vi "Close.vi"(8 "error in (no error)":errorcluster, 11 "Diode IV in":refnum<class "Diode IV.lvclass">) -> (0 "error out":errorcluster, 3 "Diode IV out":refnum<class "Diode IV.lvclass">)   [LabVIEW 2015, in "Diode Characterization.lvlib" / "Diode IV.lvclass"]
uses:
  Diode IV.lvclass
  <userlib>/Common Components/Measurement Actor/Measurement.lvclass
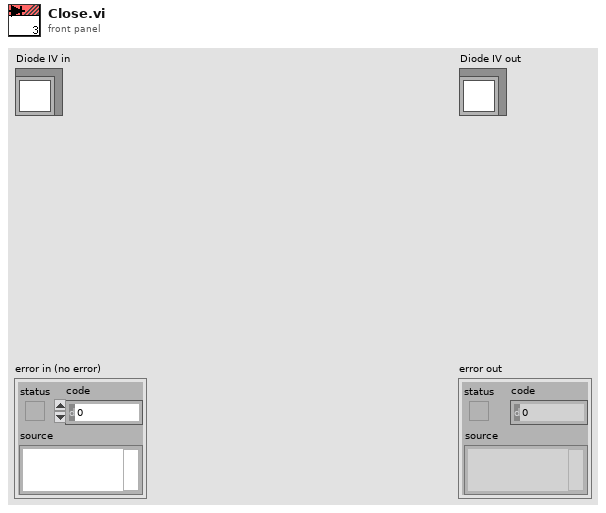
[diagram p1: front panel]
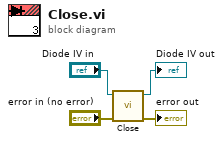
[diagram p0: block diagram]
diagram:
  n1 = call-parent "Close.vi"("error in (no error)"="error in (no error)", "Measurement in"="Diode IV in") -> ("error out"=→"error out":errorcluster, "Measurement out"=→"Diode IV out":refnum<class "Diode IV.lvclass">)  [unwired: 8 in]
